vi "Add File Error Core.vi"(8 "error in (no error)":errorcluster, 10 "String to Append":string, 11 "Error":T1) -> (0 "error out":errorcluster)   [LabVIEW 2021, in "File_CIF_U.lvlib"]
uses:
  File_CIF_U.lvlib
  typedef/File Errors.ctl
  Errors/Errors_CIF_U.lvlib
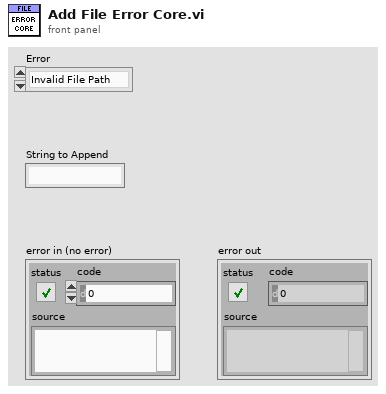
[diagram p1: front panel]
types:
  T1 = typedef "File_CIF_U.lvlib/File Errors.ctl" = enum16{"Invalid File Path"}
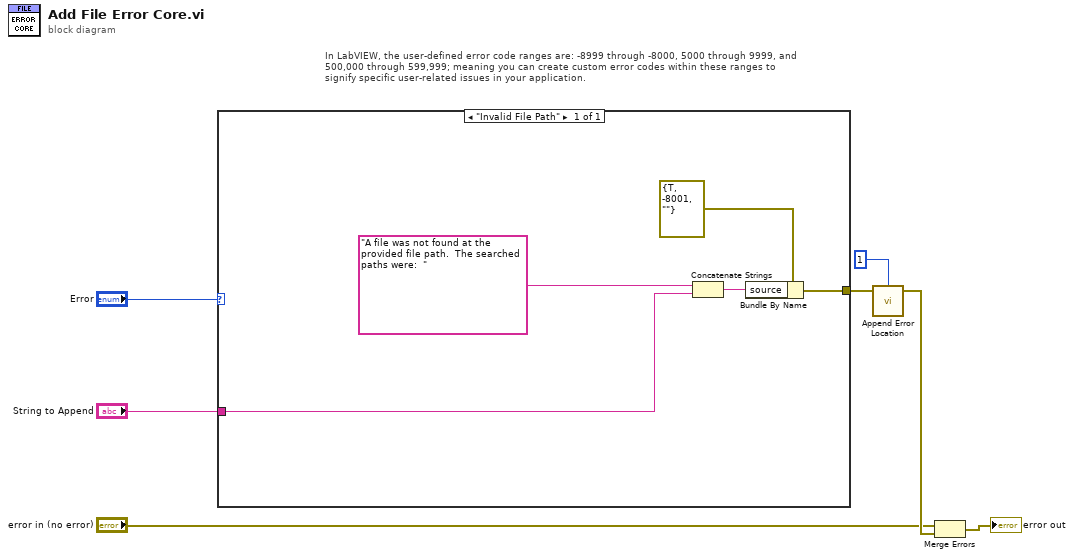
[diagram p0: block diagram]
diagram:
  # "In LabVIEW, the user-defined error code ranges are: -8999 through -8000, 5000 through 9999, and 500,000 through 599,999; meaning you can create custom error codes within these ranges to signify specific user-related issues in your application."
  n1 = case shown="\"Invalid File Path\"" "Error" {
    tunnel: "String to Append" -> [w9]
    tunnel: [w11] -> w6
    frame "Invalid File Path" {
      n2 = Concatenate Strings("A file was not found at the provided file path.  The searched paths were:  " ("source"), w9) -> (w8:string)
      n3 = Bundle By Name(cluster=errorcluster {"status"=TRUE, "code"=-8001, "source"=""} ("Invalid ID"), "source"=w8) -> (w11:errorcluster)
    }
  }
  n4 = call "Append Error Location.vi"("error in (no error)"=w6, "Chain Depth"=1) -> ("error out"=w7:errorcluster)  [unwired: 3 in]
  n5 = Merge Errors("error in (no error)", w7) -> (→"error out":errorcluster)
